vi "PMOD Example(FPGA).vi"() -> ()   [LabVIEW 2014]
uses:
  Controls/SPIExample.CurrentStateFPGA.ctl
  <userlib>/_NI SPI IP/FPGA/Controllers/Public/Spi Master Outputs.ctl
  <userlib>/_NI SPI IP/FPGA/Controllers/Public/Transfer Settings.ctl
  <vilib>/SPIAPI/DIO/SPI DIO Enable Lines.ctl
  <vilib>/SPIAPI/DIO/SPI Digital IO Lines.ctl
  <vilib>/Platform/TimedLoop/XDataNode/timing_clust.ctl
  <vilib>/Platform/TimedLoop/XDataNode/nitl_modes.ctl
  <vilib>/Platform/TimedLoop/XDataNode/wakeup.ctl
  <vilib>/rvi/Emulation/niFpgaGetClockAttributes.vi
  <vilib>/rvi/Emulation/niFpgaSctlEmulationGetInTimedLoop.vi
  <vilib>/rvi/Emulation/niFpgaEmulationReportErrorSimple.vi
  <vilib>/rvi/Emulation/niFpgaProcessEmulError.vi
  <vilib>/rvi/Emulation/niFpgaCriticalErrorInLSC.vi
  <vilib>/rvi/interface/RandomDataEmulation/niFpgaRandomDataHandleErrors.vi
  <vilib>/Platform/TimedLoop/XDataNode/XDataNode.xnode
  <vilib>/rvi/DataTransferAndStorage/Container/XNode/niFpgaContainer.xnode
  <vilib>/rvi/interface/RandomDataEmulation/nirviRandomDataFpgaReadWriteTemplate.vi
  <vilib>/Platform/TimedLoop/XDataNode/XDNodeRunTimeDep.lvlib
  <userlib>/_NI SPI IP/FPGA/Controllers/NI SPI IP (FPGA).lvlib
panel:
  out "Raw ADC Data":u64
  out "read Iterations":i32
  in  "Data To ADC":u64=2147483648
  in  "Chip Select":u8
  in  "SPI PHY Settings":T1={"Divide Value"=20, "Transfer Length (bits)"=32, "CS Asserted Polarity"=FALSE, "Clock Polarity (CPOL)"=FALSE, "Clock Phase (CPHA)"=FALSE, "Lengthen MISO Setup"=FALSE, "Direction Change Bit"=0, "MOSI Starts as Output"=FALSE, "Tristatable MOSI"=FALSE} {"Direction Change Bit" max=64 step=1; "Transfer Length (bits)" min=1 max=64 step=1}
  out "spi output":T2
  in  "Chan Offset Array":sgl[](array[numeric])=[0.0, 0.0, 0.0, 0.0, 0.0, 0.0, 0.0, 0.0, 0.0, 0.0, 0.0, 0.0, 0.0, 0.0, 0.0, 0.0, 0.0, 0.0, 0.0, 0.0, 0.0, 0.0, 0.0, 0.0, 0.0, 0.0, 0.0, 0.0, 0.0, 0.0, 0.0, 0.0, 0.0, 0.0, 0.0, 0.0, 0.0, 0.0, 0.0, 0.0]
  out "SGL Data":sgl
  out "State":T3
  out "Iterations":i32
  in  "Debug":bool=TRUE
  out "Chan Count":bool
  out "oclk mult":u32
  in  "data rate (S/s)":u32=10000
  out "oclk freq":u32
  out "oclk div":u32
  in  "Chan Scale Array":sgl[](array[numeric])=[1.0, 1.0, 1.0, 0.0, 0.0, 0.0, 0.0, 0.0, 0.0, 0.0, 0.0, 0.0, 0.0, 0.0, 0.0, 0.0, 0.0, 0.0, 0.0, 0.0, 0.0, 0.0, 0.0, 0.0, 0.0, 0.0, 0.0, 0.0, 0.0, 0.0, 0.0, 0.0, 0.0, 0.0, 0.0, 0.0, 0.0, 0.0, 0.0, 0.0]
  out "FPGA Error":errorcluster
  out "Finished":bool
  in  "stop":bool
  out "Module Underflow":bool
  out "Acq Loop Ticks":u32
  out "DMA FIFO Full":bool
  out "First Read":bool
  in  "Number of Channels":i32=4
  in  "Acquisition Type":enum16{"Finite Samples", "Continuous Samples"}(ring)=enum."Continuous Samples"
  in  "Samps per Chan [Finite]":i32=5120
  # "OUTPUT"
  # "INPUT"
  # "ADC Data::Debug"
  # "Acquisition Parameters"
  # "SPI PHY Settings"
  # "Debug"
  # "Status"
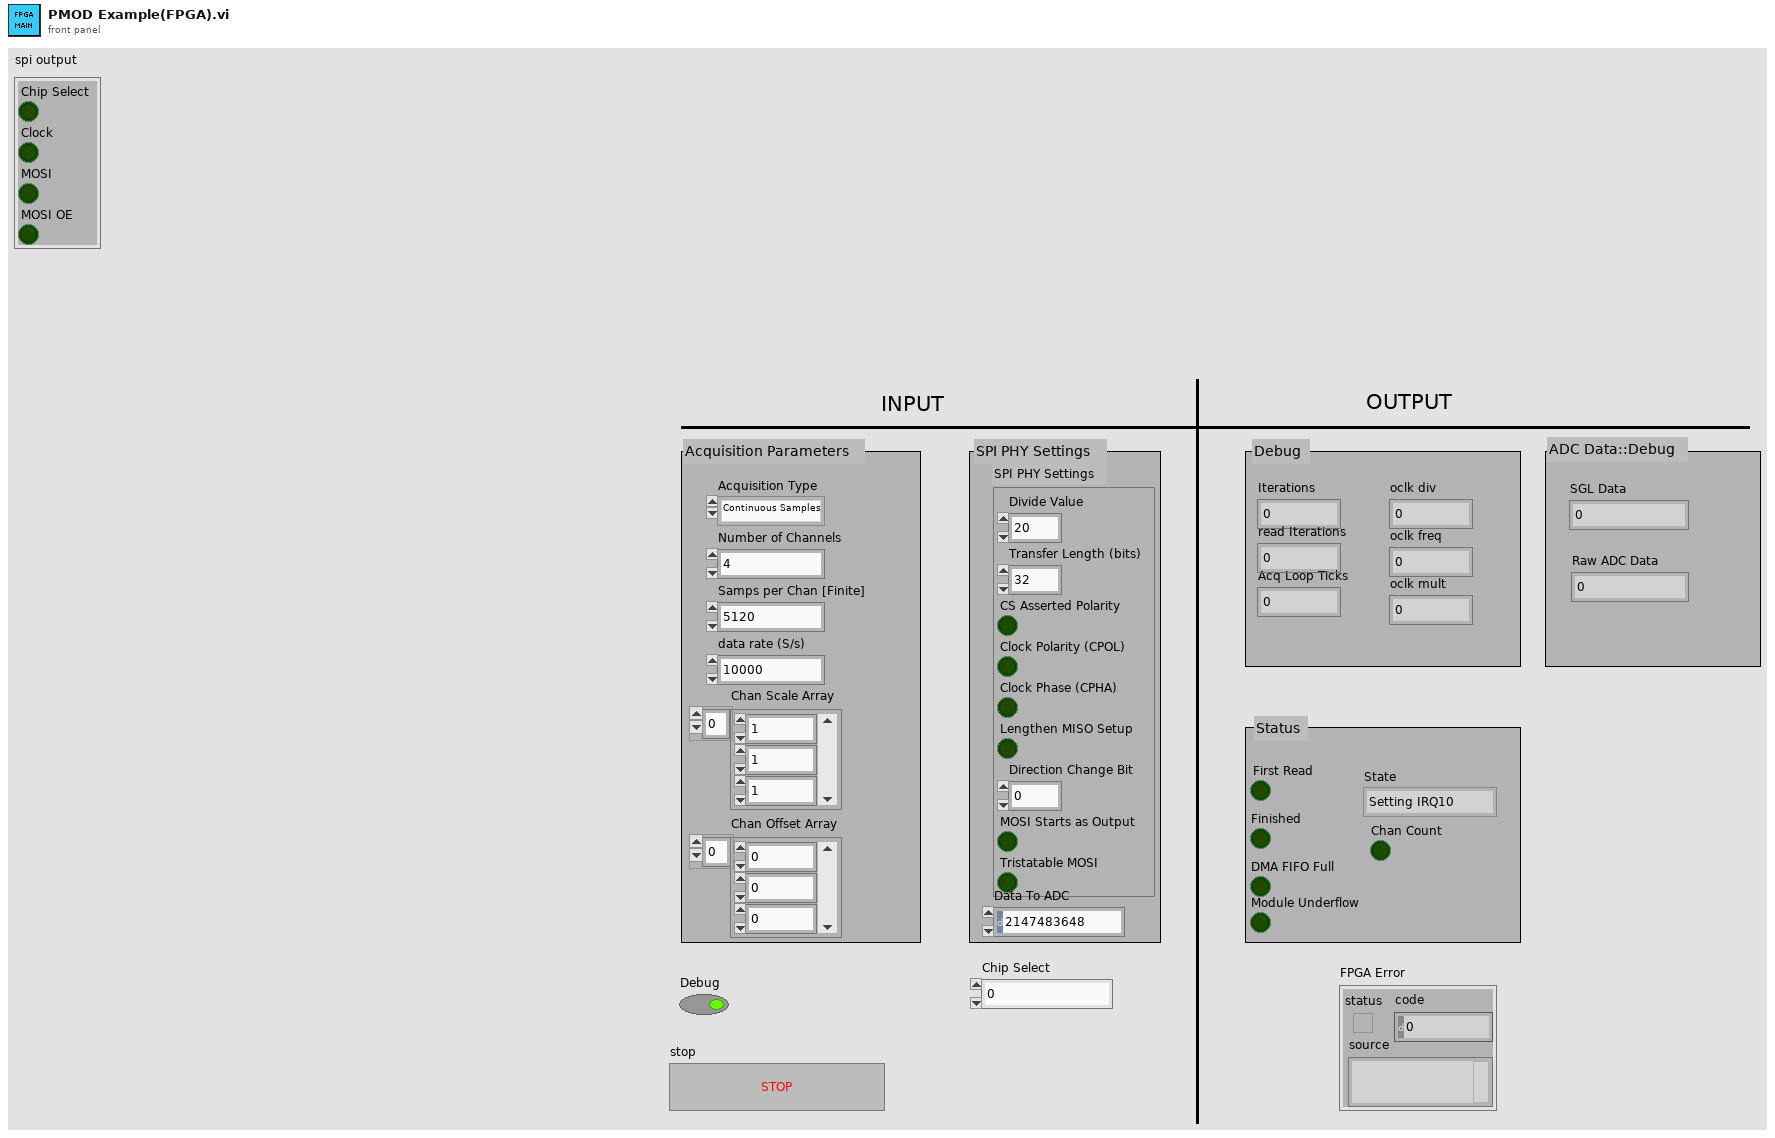
[diagram p1: front panel]
types:
  T1 = typedef "NI SPI IP (FPGA).lvlib/Transfer Settings.ctl" = cluster{"Divide Value":u8, "Transfer Length (bits)":u8, "CS Asserted Polarity":bool, "Clock Polarity (CPOL)":bool, "Clock Phase (CPHA)":bool, "Lengthen MISO Setup":bool, "Direction Change Bit":u8, "MOSI Starts as Output":bool, "Tristatable MOSI":bool}
  T2 = typedef "NI SPI IP (FPGA).lvlib/Spi Master Outputs.ctl" = cluster{"Chip Select":bool, "Clock":bool, "MOSI":bool, "MOSI OE":bool}
  T3 = typedef "SPIExample.CurrentStateFPGA.ctl" = enum16{"Setting IRQ10", "Config SPI", "Setting IRQ11", "Init Var", "IO Engine Running"}
  T4 = typedef "SPI DIO Enable Lines.ctl" = cluster{"SCLK_en":refnum<k21>, "MISO_en":refnum<k21>, "MOSI_en":refnum<k21>, "CS0_en":refnum<k21>, "CS1_en":refnum<k21>, "CS2_en":refnum<k21>, "CS3_en":refnum<k21>, "CS4_en":refnum<k21>, "CS5_en":refnum<k21>}
  T5 = typedef "SPI Digital IO Lines.ctl" = cluster{"SCLK":refnum<k21>, "MISO":refnum<k21>, "MOSI":refnum<k21>, "CS 0":refnum<k21>, "CS 1":refnum<k21>, "CS 2":refnum<k21>, "CS 3":refnum<k21>, "CS 4":refnum<k21>, "CS 5":refnum<k21>}
  T6 = typedef "XDNodeRunTimeDep.lvlib/timing_clust.ctl" = cluster{"Expected End [f-1]":u64, "Actual End [f-1]":u64, "Finished Late? [f-1]":bool, "Expected End [i-1]":u64, "Actual End [i-1]":u64, "Finished Late? [i-1]":bool, "Expected Start [i]":u64, "Actual Start [i]":u64, "Expected Start [f]":u64, "Actual Start [f]":u64, "Source Name":string, "Structure Name":string, "Period":i64, "Deadline":i64, "Offset":i64, "Start":i64, "Priority":i32, "Timeout":i32, "Mode":T7, "Wakeup Reason":T8, "Error":errorcluster, "Source Type":string, "Secondary Source Type":string, "Global End Time":u64, "Global Start Time":u64, "Frame Duration":u64, "Iteration Duration":u64, "Assigned CPU":i32, "I/O Scan Engine Mode":u32}
  T7 = typedef "XDNodeRunTimeDep.lvlib/nitl_modes.ctl" = enum32{"No Change", "Process missed periods, maintain original phase", "Discard missed periods, maintain original phase", "Process missed periods, ignore original phase", "Discard missed periods, ignore original phase"}
  T8 = typedef "XDNodeRunTimeDep.lvlib/wakeup.ctl" = enum32{"Normal", "Aborted", "Asynchronous wakeup", "Timing source error", "Timed loop error", "Timeout"}
  T9 = typedef "Internal Data (SPI API).ctl" = cluster{"DLU To SPI Engine Data FIFO":refnum<k21>, "SPI Engine to DLU Data FIFO":refnum<k21>, "Data to SPI Engine (Cache) Register":refnum<k21>, "SPI PHY Settings to SPI Engine (Cahche) Register":refnum<k21>}
  T10 = typedef "SPI Response Information.ctl" = cluster{"Data to Node":u64, "Node Id":u16}
  T11 = typedef "NI SPI IP (FPGA).lvlib/Spi Master Inputs.ctl" = cluster{"MISO":bool}
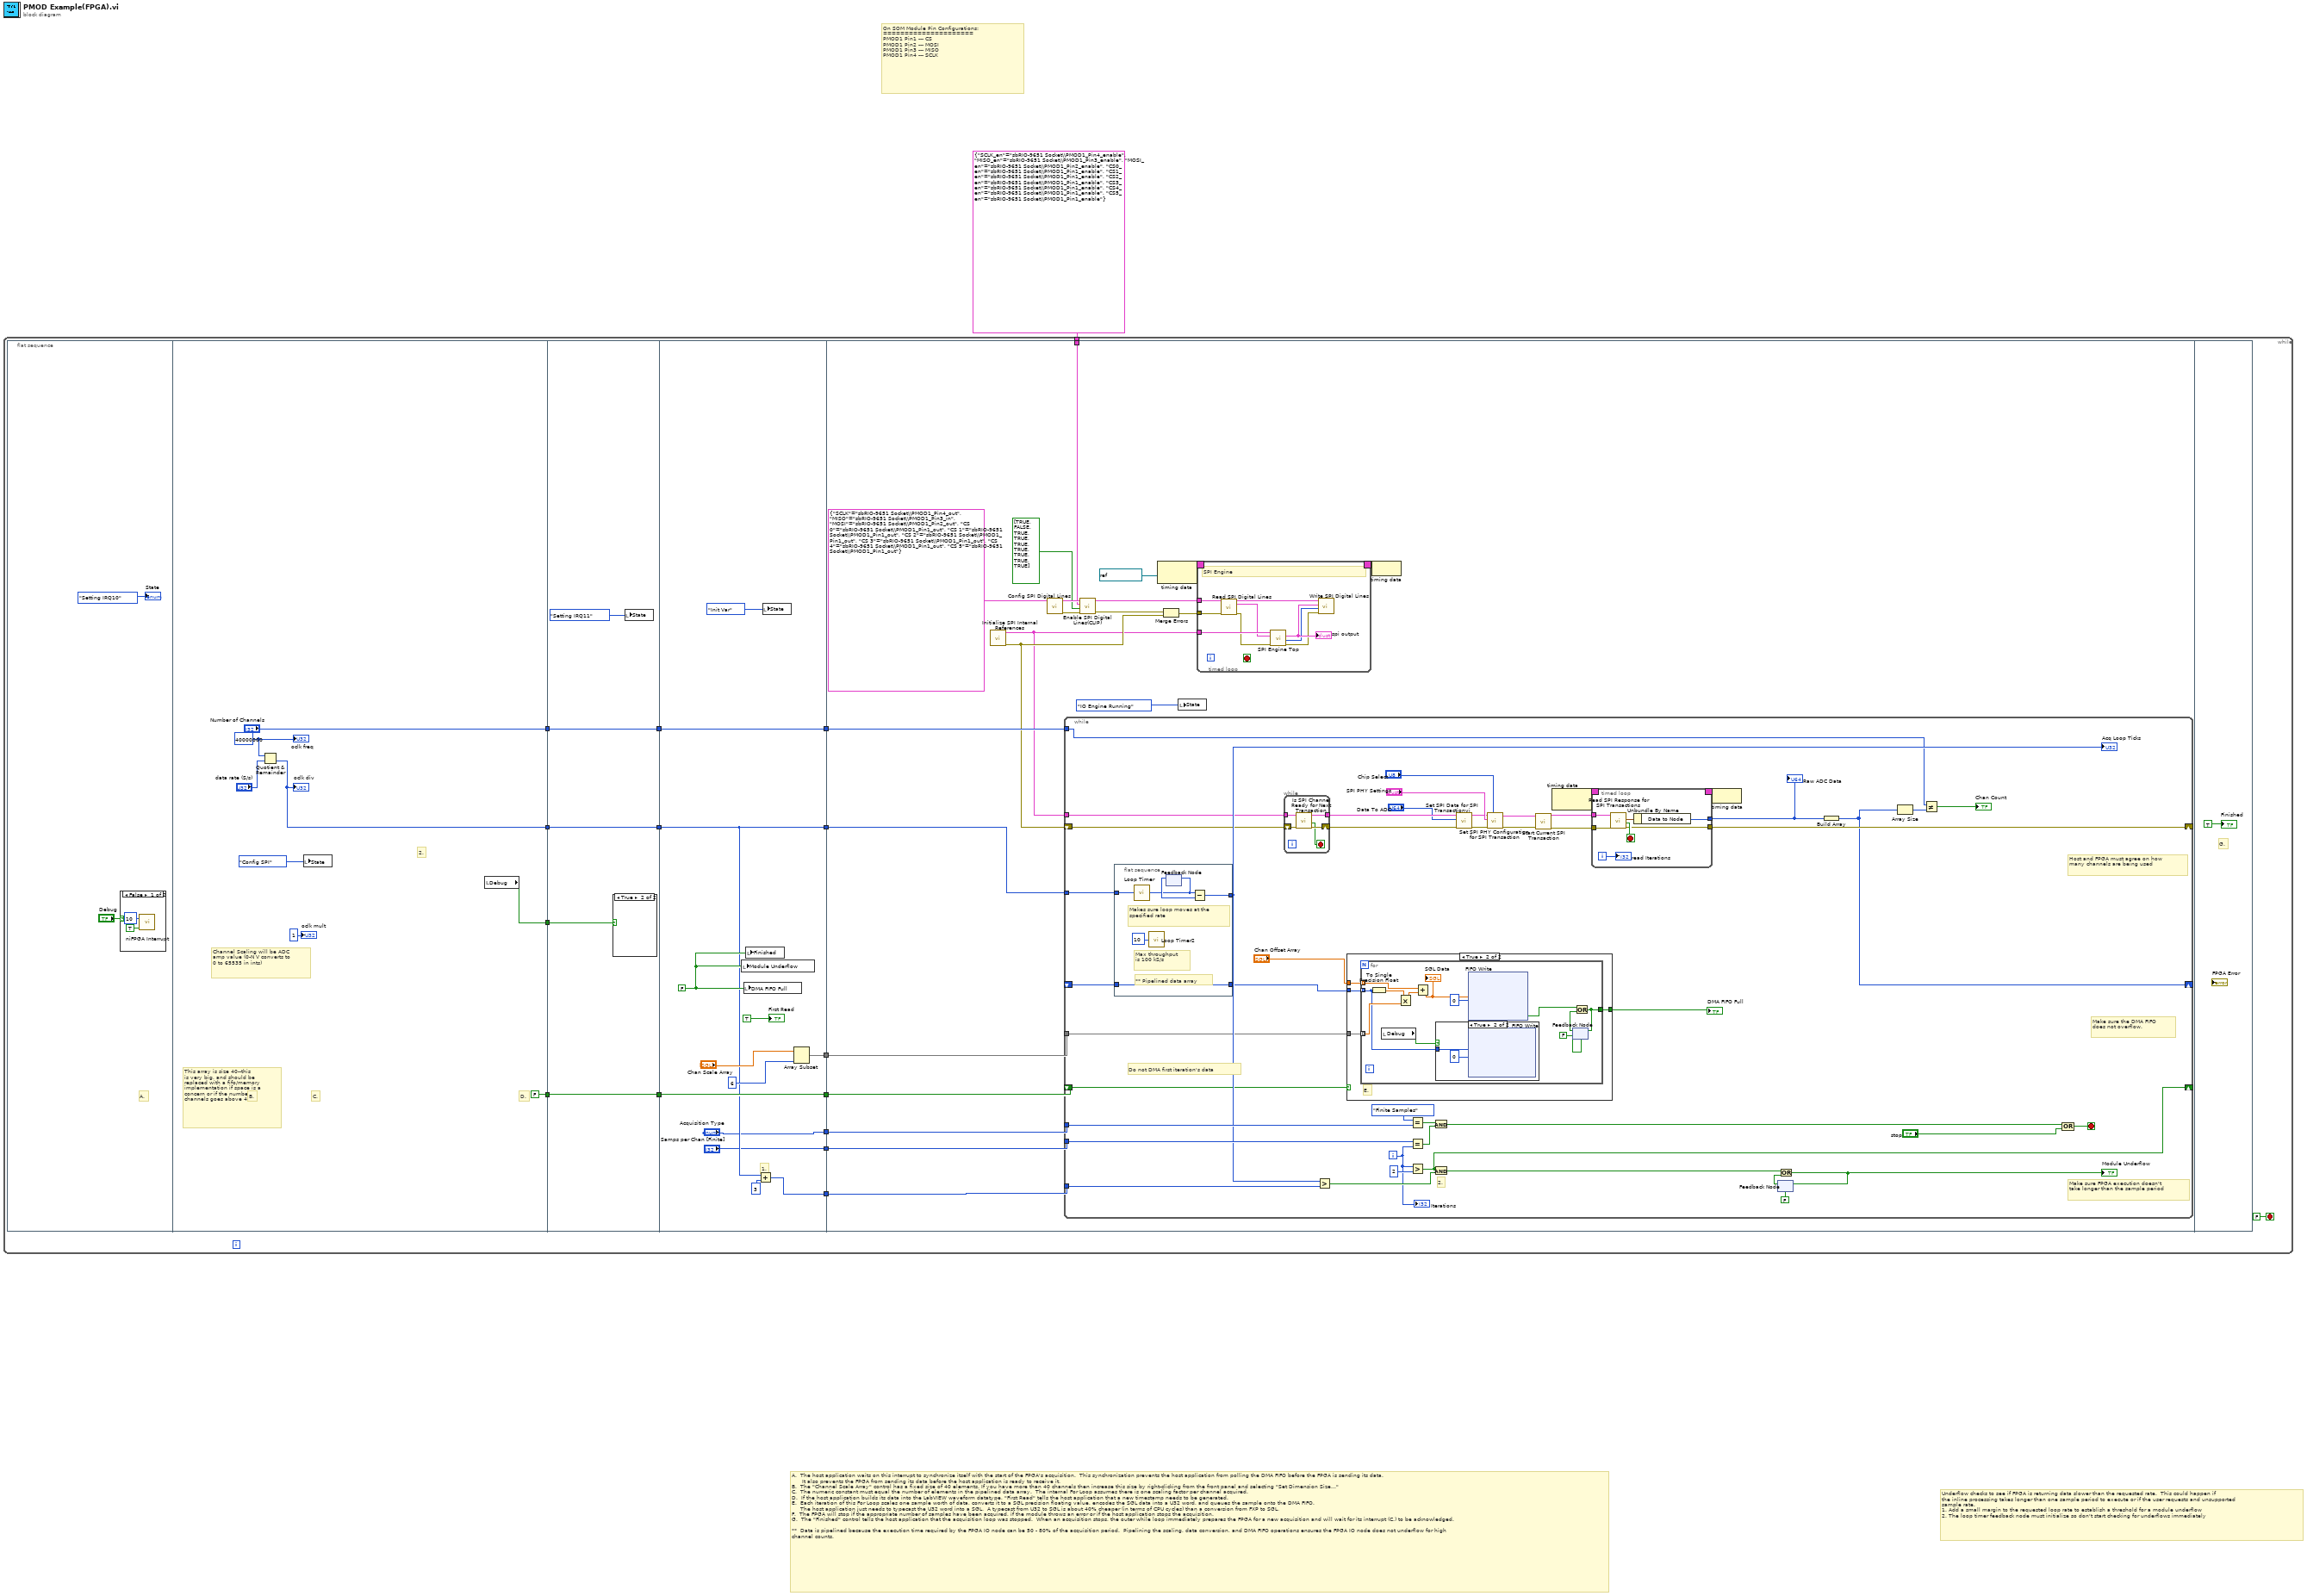
[diagram p0: block diagram]
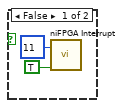
[diagram p3: hidden frame]
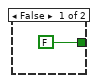
[diagram p4: hidden frame]
diagram:
  # "On SOM Module Pin Configurations:\n=====================\nPMOD1 Pin1 --- CS\nPMOD1 Pin2 --- MOSI\nPMOD1 Pin3 --- MISO\nPMOD1 Pin4 --- SCLK"
  # "Underflow checks to see if FPGA is returning data slower than the requested rate.  This could happen if\nthe inline processing takes longer than one sample period to execute or if the user requests and unsupported\nsample rate.\n1. Add a small margin to the requested loop rate to establish a threshold for a module underflow \n2. The loop timer feedback node must initialize so don't start checking for underflows immediately"
  # "A.  The host application waits on this interrupt to synchronize itself with the start of the FPGA's acquisition.  This synchronization prevents the host application from polling the DMA FIFO before the FPGA is sending its data.\n      It also prevents the FPGA from sending its data before the host application is ready to receive it.\nB.  The \"Channel Scale Array\" control has a fixed size of 40 elements. If you have more than 40 channels then increase this size by right-clicking from the front panel and selecting \"Set Dimension Size...\"\nC.  The numeric constant must equal the number of elements in the pipelined data array.  The internal For Loop assumes there is one scaling factor per channel acquired.\nD.  If the host application builds its data into the LabVIEW waveform datatype, \"First Read\" tells the host application that a new timestamp needs to be generated.\nE.  Each iteration of this For Loop scales one sample worth of data, converts it to a SGL precision floating value, encodes the SGL data into a U32 word, and queues the sample onto the DMA FIFO.  \n     The host application just needs to typecast the U32 word into a SGL.  A typecast from U32 to SGL is about 40% cheaper (in terms of CPU cycles) than a conversion from FXP to SGL.\nF.  The FPGA will stop if the appropriate number of samples have been acquired, if the module throws an error or if the host application stops the acquisition.  \nG.  The \"Finished\" control tells the host application that the acquisition loop was stopped.  When an acquisition stops, the outer while loop immediately prepares the FPGA for a new acquisition and will wait for its interrupt (C.) to be acknowledged. \n\n**  Data is pipelined because the execution time required by the FPGA IO node can be 50 - 80% of the acquisition period.  Pipelining the scaling, data conversion, and DMA FIFO operations ensures the FPGA IO node does not underflow for high\nchannel counts."
  n1 = while {
    tunnel: T4 {"SCLK_en"="sbRIO-9651 Socket\\PMOD1_Pin4_enable", "MISO_en"="sbRIO-9651 Socket\\PMOD1_Pin3_enable", "MOSI_en"="sbRIO-9651 Socket\\PMOD1_Pin2_enable", "CS0_en"="sbRIO-9651 Socket\\PMOD1_Pin1_enable", "CS1_en"="sbRIO-9651 Socket\\PMOD1_Pin1_enable", "CS2_en"="sbRIO-9651 Socket\\PMOD1_Pin1_enable", "CS3_en"="sbRIO-9651 Socket\\PMOD1_Pin1_enable", "CS4_en"="sbRIO-9651 Socket\\PMOD1_Pin1_enable", "CS5_en"="sbRIO-9651 Socket\\PMOD1_Pin1_enable"} ("Enable Lines") -> [w2]
    stop <- FALSE stop-if-true
    n2 = flat-sequence {
      tunnel: ["Number of Channels"] -> w16
      tunnel: [FALSE] -> w15
      tunnel: [w25] -> w14
      tunnel: [w23] -> w3
      tunnel: w16 -> [w34]
      tunnel: [w34] -> w13
      tunnel: w15 -> [w33]
      tunnel: [w33] -> w7
      tunnel: w14 -> [w32]
      tunnel: [w32] -> w5
      tunnel: w3 -> [w31]
      tunnel: w13 -> [w49]
      tunnel: [w49] -> w12
      tunnel: [w45] -> w11
      tunnel: ["Acquisition Type"] -> w10
      tunnel: ["Samps per Chan [Finite]"] -> w9
      tunnel: [w41] -> w8
      tunnel: w7 -> [w48]
      tunnel: [w48] -> w6
      tunnel: w5 -> [w40]
      tunnel: [w40] -> w4
      tunnel: w12 -> [w70]
      tunnel: w11 -> [w68]
      tunnel: w10 -> [w67]
      tunnel: w9 -> [w66]
      tunnel: w8 -> [w65]
      tunnel: w6 -> [w64]
      tunnel: w4 -> [w69]
      tunnel: w2 -> [w51]
      frame #0 {
        # "A."
        n3 = case shown="False" "Debug" {
          frame False {
            n4 = call <vilib>:"niFPGA Interrupt.vi"("Wait Until Cleared (F)"=TRUE ("Wait Until Cleared"), "IRQ Number (0)"=u8 10 ("IRQ Number")) -> ()  [unwired: 1 in]
          }
          frame True {
          }
        }
        "State" <- SPIExample.CurrentStateFPGA."Setting IRQ10" ("State")
      }
      frame #1 {
        w26 = u32 40000000 ("oclk freq")
        # "2."
        # "This array is size 40--this\nis very big, and should be\nreplaced with a fifo/memory\nimplementation if space is a\nconcern or if the number of \nchannels goes above 40"
        # "Channel Scaling will be ADC\namp value (0-N V converts to\n0 to 65535 in ints)"
        # "D."
        # "C."
        # "B."
        n5 = Quotient & Remainder(x=w26, y="data rate (S/s)") -> (floor(x/y)=w25:u32)  [unwired: 1 out]
        "oclk div" <- w25
        n6 = local write "State"(SPIExample.CurrentStateFPGA."Config SPI" ("State")) -> ()
        n7 = local read "Debug"() -> (w23:bool)
        "oclk freq" <- w26
        "oclk mult" <- u32 1 ("oclk mult")
      }
      frame #2 {
        n8 = case shown="True" w31 {
          frame False {
            n9 = call <vilib>:"niFPGA Interrupt.vi"("Wait Until Cleared (F)"=TRUE ("Wait Until Cleared"), "IRQ Number (0)"=u8 11 ("IRQ Number")) -> ()  [unwired: 1 in]
          }
          frame True {
          }
        }
        n10 = local write "State"(SPIExample.CurrentStateFPGA."Setting IRQ11" ("State")) -> ()
      }
      frame #3 {
        w47 = FALSE ("Module Underflow")
        # "1."
        n11 = local write "Module Underflow"(w47) -> ()
        n12 = local write "DMA FIFO Full"(w47) -> ()
        n13 = local write "Finished"(w47) -> ()
        n14 = Add(x=w40, y=u32 3) -> (x+y=w41:u32)
        n15 = local write "State"(SPIExample.CurrentStateFPGA."Init Var" ("State")) -> ()
        n16 = Array Subset(array="Chan Scale Array", length=6) -> (w45:sgl[])  [unwired: 1 in]
        "First Read" <- TRUE ("First Read")
      }
      frame #4 {
        n17 = call <vilib>:"Initialize SPI Internal References.vi"() -> ("error out"=w62:errorcluster, "SPI API References"=w61:T9)  [unwired: 10 in]
        n18 = call <vilib>:"Config SPI Digital Lines.vi"("SPI DIO Lines"=T5 {"SCLK"="sbRIO-9651 Socket\\PMOD1_Pin4_out", "MISO"="sbRIO-9651 Socket\\PMOD1_Pin3_in", "MOSI"="sbRIO-9651 Socket\\PMOD1_Pin2_out", "CS 0"="sbRIO-9651 Socket\\PMOD1_Pin1_out", "CS 1"="sbRIO-9651 Socket\\PMOD1_Pin1_out", "CS 2"="sbRIO-9651 Socket\\PMOD1_Pin1_out", "CS 3"="sbRIO-9651 Socket\\PMOD1_Pin1_out", "CS 4"="sbRIO-9651 Socket\\PMOD1_Pin1_out", "CS 5"="sbRIO-9651 Socket\\PMOD1_Pin1_out"} ("Chip Select DIO Lines")) -> ("error out"=w53:errorcluster, "Chip Select DIO Lines"=w54:T5)  [unwired: 9 in]
        n19 = while {
          tunnel: w67 -> [w127]
          tunnel: w66 -> [w126]
          shift-right: [w97] -> _
          shift-left: _ -> [w120]
          tunnel: w70 -> [w105]
          tunnel: w69 -> [w125]
          tunnel: w65 -> [w122]
          tunnel: w68 -> [w110]
          shift-right: [w109] -> _
          shift-left: w64 -> [w119]
          shift-right: [w99] -> _
          shift-left: w62 -> [w100]
          tunnel: w61 -> [w101]
          i -> [w118]
          stop <- w129 stop-if-true
          # "2."
          # "Do not DMA first iteration's data"
          # "Host and FPGA must agree on how \nmany channels are being used"
          # "Make sure the DMA FIFO\ndoes not overflow."
          # "Make sure FPGA execution doesn't\ntake longer than the sample period"
          n20 = flat-sequence {
            tunnel: w125 -> [w172]
            tunnel: [w169] -> w121
            tunnel: [w168] -> w108
            tunnel: w120 -> [w168]
            frame #0 {
              # "Max throughput\nis 100 kS/s"
              # "Makes sure loop moves at the\nspecified rate"
              # "** Pipelined data array"
              n21 = call "Loop Timer"("Count(Ticks)"=w172) -> ("Tick Count(Ticks)"=w170:u32)
              n22 = call "Loop Timer2"("Count(uSec)"=u8 10 ("Count(Ticks)")) -> ()  [unwired: 1 out]
              n23 = feedback-in #1(w170) -> ()
              n24 = feedback #1() -> (w171:u32)  [unwired: 1 out]
              n25 = Subtract(x=w170, y=w171) -> (x-y=w169:u32)
            }
          }
          n26 = while {
            shift-right: [w136] -> w103
            shift-left: w100 -> [w133]
            tunnel: w101 -> [w134]
            tunnel: [w135] -> w102
            stop <- w132 stop-if-true
            n27 = call <vilib>:"Is SPI Channel Ready for Next Transaction.vi"("error in"=w133, "Private Data In"=w134) -> ("error out"=w136:errorcluster, "SPI Channel Ready"=w132:bool, "Private Data Out"=w135:T9)  [unwired: 6 in, 1 out]
          }
          n28 = Greater?(x=w121, y=w122) -> (0:w124:bool)
          n29 = case shown="True" w119 {
            tunnel: [FALSE w152] -> w128
            tunnel: w108 -> [_ w151]
            tunnel: w110 -> [_ w150]
            tunnel: "Chan Offset Array" -> [_ w149]
            frame False {
            }
            frame True {
              # "E."
              n30 = for {
                tunnel: [w161] -> w152
                tunnel: w151 -> [w153] mode=indexing
                tunnel: w150 -> [w159] mode=indexing
                tunnel: w149 -> [w154] mode=indexing
                n31 = To Single Precision Float(number=w153) -> (single precision float=w157:sgl)
                n32 = local read "Debug"() -> (w156:bool)
                n33 = Multiply(x=w157, y=w159) -> (x*y=w158:sgl)
                n34 = Add(x=w154, y=w158) -> (x+y=w155:sgl)
                "SGL Data" <- w155
                n35 = case shown="True" w156 {
                  tunnel: w153 -> [_ w165]
                  frame False {
                  }
                  frame True {
                    n36 = xnode ("FIFO Write")("Element"=w165, "Timeout"=0) -> ()  [unwired: 1 in, 2 out]
                  }
                }
                n37 = xnode ("FIFO Write")("Element"=w155, "Timeout"=0) -> ("Timed Out?"=w164:bool)  [unwired: 1 in, 1 out]
                n38 = feedback #2(FALSE) -> (w162:bool)
                n39 = Or(x=w164, y=w162) -> (x .or. y?=w161:bool)
                n40 = feedback-in #2(w161) -> ()
              }
            }
          }
          "DMA FIFO Full" <- w128
          n41 = Equal?(x=enum16{"Finite Samples", "Continuous Samples"}."Finite Samples" ("y"), y=w127) -> (x = y?=w113:bool)
          n42 = Equal?(x=w126, y=w118) -> (x = y?=w112:bool)
          n43 = Greater?(x=w118, y=2) -> (0:w109:bool)
          n44 = And(x=w113, y=w112) -> (x .and. y?=w111:bool)
          n45 = And(x=w109, y=w124) -> (x .and. y?=w115:bool)
          n46 = call <vilib>:"Set SPI Data for SPI Transactionvi.vi"("error in"=w103, "Data In"="Data To ADC", "Private Data In"=w102) -> ("error out"=w91:errorcluster, "Private Data Out"=w92:T9)  [unwired: 7 in]
          n47 = call <vilib>:"Set SPI PHY Configuration for SPI Transaction.vi"("Chip Select"="Chip Select", "error in"=w91, "SPI PHY Settings"="SPI PHY Settings", "Private Data In"=w92) -> ("error out"=w88:errorcluster, "Private Data Out"=w89:T9)  [unwired: 6 in]
          n48 = call <vilib>:"Start Current SPI Transaction.vi"("error in"=w88, "Private Data In"=w89) -> ("error out"=w93:errorcluster, "Private Data Out"=w87:T9)  [unwired: 7 in, 1 out]
          n49 = node-c288() -> (w96:T6)  [unwired: 1 in]
          n50 = timed-loop {
            timing: w96 -> [_]
            timing-out: [_] -> w95
            tunnel: w93 -> [w143]
            tunnel: w87 -> [w142]
            tunnel: [w137] -> w98
            tunnel: [w139] -> w99
            i -> [w138]
            stop <- w141 stop-if-true
            n51 = call <vilib>:"Read SPI Response for SPI Transactions.vi"("error in"=w143, "Private Data In"=w142) -> ("error out"=w139:errorcluster, "Read Data Valid?"=w141:bool, "Read Data"=w140:T10)  [unwired: 6 in, 1 out]
            n52 = Unbundle By Name(w140) -> ("Data to Node"=w137:u64)
            "read Iterations" <- w138
          }
          "Raw ADC Data" <- w98
          n53 = node-c288(w95) -> ()
          n54 = feedback #3(FALSE) -> (w117:bool)
          n55 = Or(x=w115, y=w117) -> (x .or. y?=w114:bool)
          "Module Underflow" <- w114
          n56 = feedback-in #3(w114) -> ()
          n57 = Build Array(w98) -> (w97:u64[])
          n58 = Array Size(array=w97) -> (size(s)=w107:i32)
          n59 = Not Equal?(x=w105, y=w107) -> (x != y?=→"Chan Count":bool)
          n60 = Compound Arithmetic op=OR(w111, "stop") -> (w129:bool)
          "Acq Loop Ticks" <- w121
          "Iterations" <- w118
        }
        n61 = call <vilib>:"Enable SPI Digital Lines(CLIP).vi"("error in"=w53, "Enable"=bool[] [TRUE, FALSE, TRUE, TRUE, TRUE, TRUE, TRUE, TRUE, TRUE], "Enable Lines"=w51, "SPI DIO Lines"=w54) -> ("error out"=w55:errorcluster, "Chip Select DIO Lines"=w56:T5)  [unwired: 6 in]
        n62 = node-c288(refnum<k21> "120MHz" ("Source Name")) -> (w60:T6)
        n63 = Merge Errors(w55, w62) -> (w58:errorcluster)
        n64 = local write "State"(SPIExample.CurrentStateFPGA."IO Engine Running" ("State")) -> ()
        n65 = timed-loop {
          tunnel: w61 -> [w76]
          tunnel: w58 -> [w74]
          tunnel: w56 -> [w78]
          timing: w60 -> [_]
          timing-out: [_] -> w59
          stop <- _ stop-if-true
          # "SPI Engine"
          n66 = call <vilib>:"Read SPI Digital Lines.vi"("Chip Select DIO Lines"=w78, "error in"=w74) -> ("Chip Select DIO Lines Out"=w79:T5, "SPI Read Data"=w75:T11, "error out"=w73:errorcluster)  [unwired: 11 in]
          n67 = call <vilib>:"SPI Engine Top.vi"("error in"=w73, "SPI Read Data"=w75, "SPI API References"=w76) -> ("error out"=w72:errorcluster, "Chip Select ID"=w71:u8, "SPI DIO Output"=w77:T2)  [unwired: 5 in, 1 out]
          "spi output" <- w77
          n68 = call <vilib>:"Write SPI Digital Lines.vi"("error in"=w72, "CS Index"=w71, "spi output"=w77, "Chip Select DIO Lines"=w79) -> ()  [unwired: 6 in, 2 out]
        }
        n69 = node-c288(w59) -> ()
      }
      frame #5 {
        # "G."
        "Finished" <- TRUE ("Finished")
      }
    }
  }
